vi "Convert Temp.vi"() -> ()   [LabVIEW 2014]
panel:
  in  "?":bool
  out "Converted Temp.":dbl
  in  "Temp.":dbl
  in  "Enum":T1(ring)
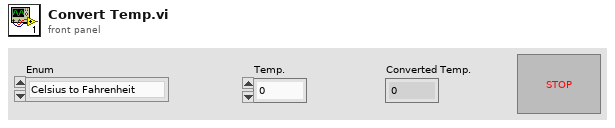
[diagram p1: front panel]
types:
  T1 = enum16{"Celsius to Fahrenheit", "Fahrenheit to Celsius", "Celsius to Kelvin", "Fahrenheit to Kelvin"}
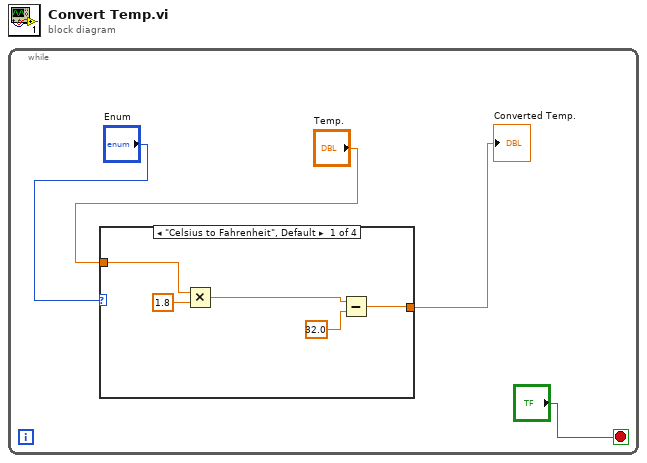
[diagram p0: block diagram]
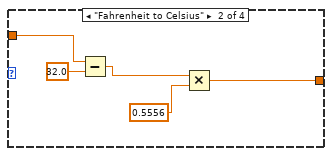
[diagram p2: hidden frame]
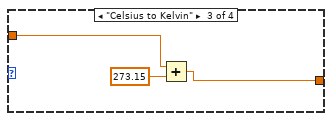
[diagram p3: hidden frame]
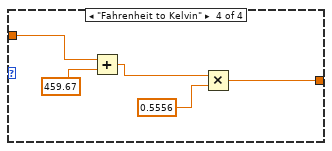
[diagram p4: hidden frame]
diagram:
  n1 = while {
    stop <- "?" stop-if-true
    n2 = case shown="\"Celsius to Fahrenheit\", Default" "Enum" {
      tunnel: "Temp." -> [w5 w13 w16 w22]
      tunnel: [w9 w10 w15 w18] -> w2
      frame "Celsius to Fahrenheit", Default {
        n3 = Multiply(x=w5, y=1.8) -> (x*y=w7:dbl)
        n4 = Subtract(x=w7, y=32.0) -> (x-y=w9:dbl)
      }
      frame "Fahrenheit to Celsius" {
        n5 = Subtract(x=w13, y=32.0) -> (x-y=w12:dbl)
        n6 = Multiply(x=w12, y=0.5556) -> (x*y=w10:dbl)
      }
      frame "Celsius to Kelvin" {
        n7 = Add(x=w16, y=273.15) -> (x+y=w15:dbl)
      }
      frame "Fahrenheit to Kelvin" {
        n8 = Add(x=w22, y=459.67) -> (x+y=w20:dbl)
        n9 = Multiply(x=w20, y=0.5556) -> (x*y=w18:dbl)
      }
    }
    "Converted Temp." <- w2
  }
